vi "Cron Weekdays.vi"(7 "Cron":refnum<class "Cron.lvclass">, 10 "Cron":T1) -> (2 "Cron Time":T1)   [LabVIEW 2013, in "openCron.lvlib" / "Cron.lvclass"]
uses:
  Cron.lvclass
  CronTime -- cluster.ctl
  Cron Interval -- enum.ctl
  Cron.lvclass/Cron.ctl
  <vilib>/LabVIEW Open Source Project/Epoch Date & Time/GregorianCal_Month -- enum.ctl
  <vilib>/LabVIEW Open Source Project/Epoch Date & Time/GregorianCal_MonthLengths.vi
  <vilib>/LabVIEW Open Source Project/Epoch Date & Time/isLeapYear (integer).vi
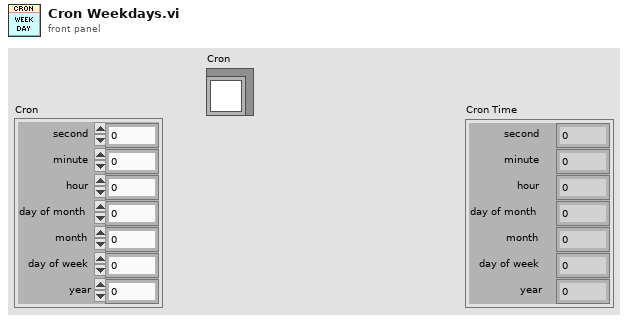
[diagram p1: front panel]
types:
  T1 = typedef "openCron.lvlib/Cron.lvclass/CronTime -- cluster.ctl" = cluster{"second":i32, "minute":i32, "hour":i32, "day of month":i32, "month":i32, "day of week":i32, "year":i32}
  T2 = typedef "openCron.lvlib/Cron.lvclass/Cron Interval -- enum.ctl" = enum16{"Seconds", "Minutes", "Hours", "Day of Month", "Month", "Day of Week", "Year"}
  T3 = typedef "openCron.lvlib/Cron.lvclass/Cron Interval -- cluster.ctl" = cluster{"Values":i32[], "All":bool, "Any":bool}
  T4 = typedef "GregorianCal_Month -- enum.ctl" = enum16{"January", "February", "March", "April", "May", "June", "July", "August", "September", "October", "November", "December"}
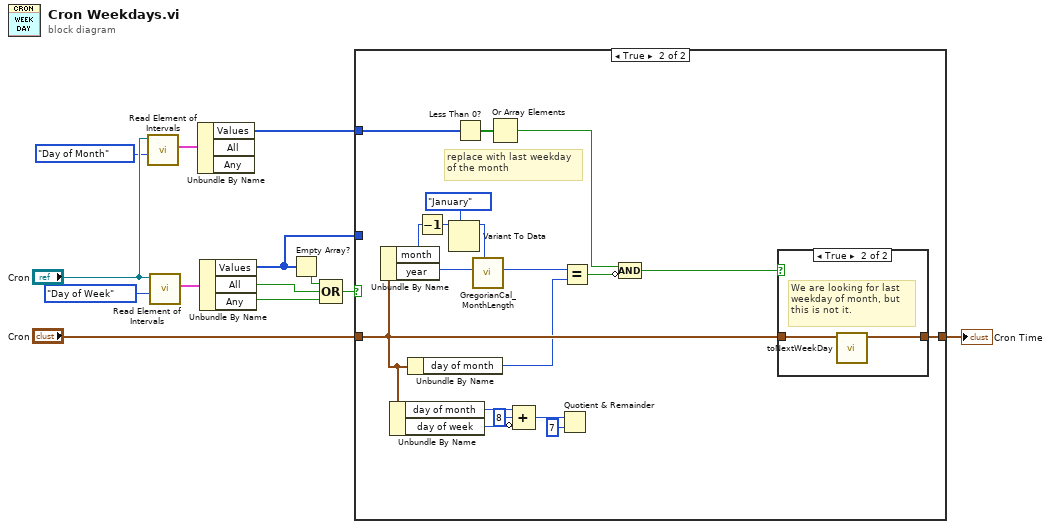
[diagram p0: block diagram]
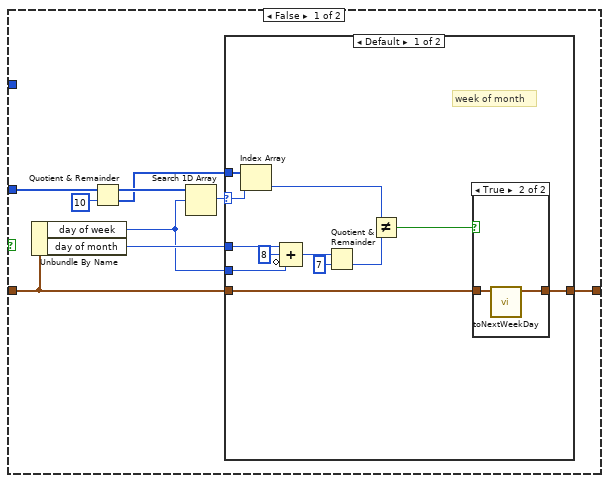
[diagram p2: hidden frame]
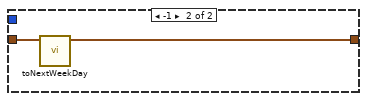
[diagram p4: hidden frame]
diagram:
  n1 = call "Read Element of Intervals.vi"("Interval"=Cron_Interval_--_enum."Day of Month", "Cron in"="Cron") -> ("Interval"=w3:T3)  [unwired: 7 in, 2 out]
  n2 = call "Read Element of Intervals.vi"("Interval"=Cron_Interval_--_enum."Day of Week", "Cron in"="Cron") -> ("Interval"=w11:T3)  [unwired: 7 in, 2 out]
  n3 = Unbundle By Name(w3) -> ("Values"=w2:i32[])  [unwired: 2 out]
  n4 = Unbundle By Name(w11) -> ("Values"=w6:i32[], "All"=w9:bool, "Any"=w10:bool)
  n5 = Empty Array?(array=w6) -> (empty?=w8:bool)
  n6 = Compound Arithmetic op=OR(w8, w9, w10) -> (w7:bool)
  n7 = case shown="True" w7 {
    tunnel: [w21 w53] -> w13
    tunnel: "Cron" -> [w22 w52]
    tunnel: w6 -> [w18 _]
    tunnel: w2 -> [_ w45]
    frame False {
      n8 = Unbundle By Name(w22) -> ("day of week"=w14:i32, "day of month"=w15:i32)
      n9 = Quotient & Remainder(x=w18, y=10) -> (x-y*floor(x/y)=w17:i32[], floor(x/y)=w16:i32[])
      n10 = Search 1D Array(1D array=w17, element=w14) -> (index of element=w20:i32)  [unwired: 1 in]
      n11 = case shown="Default" w20 {
        selector: w20 -> [w34 _]
        tunnel: w22 -> [w27 w39]
        tunnel: [w33 w38] -> w21
        tunnel: w16 -> [w24 _]
        tunnel: w15 -> [w26 _]
        tunnel: w14 -> [w25 _]
        frame Default {
          # "week of month"
          n12 = Index Array(array=w24, index=w34) -> (element=w28:i32)
          n13 = Compound Arithmetic op=ADD(w26, 8 ("value"), invert w25) -> (w29:i32)
          n14 = Quotient & Remainder(x=w29, y=7) -> (floor(x/y)=w31:i32)  [unwired: 1 out]
          n15 = Not Equal?(x=w28, y=w31) -> (x != y?=w23:bool)
          n16 = case shown="True" w23 {
            tunnel: w27 -> [w35 w37]
            tunnel: [w35 w36] -> w33
            frame False {
            }
            frame True {
              n17 = call "toNextWeekDay.vi"("Cron in"=w37) -> ("Cron out"=w36:T1)  [unwired: 10 in]
            }
          }
        }
        frame -1 {
          n18 = call "toNextWeekDay.vi"("Cron in"=w39) -> ("Cron out"=w38:T1)  [unwired: 10 in]
        }
      }
    }
    frame True {
      # "replace with last weekday\nof the month"
      n19 = Unbundle By Name(w52) -> ("month"=w55:i32, "year"=w54:i32)
      n20 = Unbundle By Name(w52) -> ("day of month"=w48:i32, "day of week"=w47:i32)
      n21 = Unbundle By Name(w52) -> ("day of month"=w46:i32)
      n22 = Decrement(x=w55) -> (x-1=w58:i32)
      n23 = Variant To Data(type=GregorianCal_Month_--_enum."January" ("Month"), Variant=w58) -> (data=w57:T4)  [unwired: 1 in, 1 out]
      n24 = Less Than 0?(x=w45) -> (x < 0?=w44:bool[])
      n25 = call <vilib>:"GregorianCal_MonthLength.vi"("Month"=w57, "Year (0: this year)"=w54) -> ("Nb Days"=w43:i32)  [unwired: 9 in]
      n26 = Or Array Elements(Boolean array=w44) -> (logical OR=w42:bool)
      n27 = Compound Arithmetic op=ADD(w48, 8 ("value"), invert w47) -> (w49:i32)
      n28 = Quotient & Remainder(x=w49, y=7) -> ()  [unwired: 2 out]
      n29 = Equal?(x=w43, y=w46) -> (x = y?=w41:bool)
      n30 = Compound Arithmetic op=AND(w42, invert w41) -> (w40:bool)
      n31 = case shown="True" w40 {
        tunnel: w52 -> [w59 w61]
        tunnel: [w59 w60] -> w53
        frame False {
        }
        frame True {
          # "We are looking for last\nweekday of month, but\nthis is not it."
          n32 = call "toNextWeekDay.vi"("Cron in"=w61) -> ("Cron out"=w60:T1)  [unwired: 10 in]
        }
      }
    }
  }
  "Cron Time" <- w13
